vi "PS Set Rate.vi"(0 "VISA Resource Name":refnum<visa-resource-name>, 1 "Old Slew Rate":dbl format="%.1f", 2 "Slew Rate [A/S]":dbl format="%.1f", 3 "error In":errorcluster) -> (4 "Slew Rate Out [A/S]":dbl format="%.1f", 5 "dup VISA Resource Name":refnum<visa-resource-name>, 7 "Update?":bool, 8 "error Out":errorcluster)   [LabVIEW 2019]
uses:
  Serial Support VISA.llb/Serial Actions.ctl
  PS Comm Globals.vi
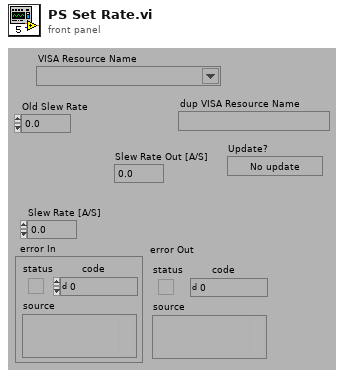
[diagram p1: front panel]
types:
  T1 = typedef "Serial Actions.ctl" = enum16{"Init", "Break", "Clear Buffer", "Write", "Read", "N Bytes", "Lock", "Unlock", "Close"}
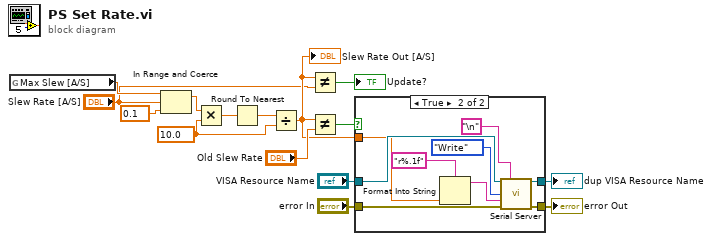
[diagram p0: block diagram]
diagram:
  w5 = 10.0 ("y")
  n1 = global read "PS Comm Globals.vi" "Max Slew [A/S]"() -> (w8:dbl)
  n2 = In Range and Coerce(upper limit=w8, x="Slew Rate [A/S]", lower limit=0.1 ("y")) -> (coerced(x)=w4:dbl)  [unwired: 1 out]
  n3 = Multiply(x=w4, y=w5) -> (x*y=w11:dbl)
  n4 = Round To Nearest(number=w11) -> (nearest integer value=w6:dbl)
  n5 = Divide(x=w6, y=w5) -> (x/y=w3:dbl)
  "Slew Rate Out [A/S]" <- w3
  n6 = Not Equal?(x=w3, y="Slew Rate [A/S]") -> (x != y?=→"Update?":bool)
  n7 = Not Equal?(x=w3, y="Old Slew Rate") -> (x != y?=w12:bool)
  n8 = case shown="True" w12 {
    tunnel: "error In" -> [w17 w26]
    tunnel: [w17 w25] -> w14
    tunnel: w3 -> [_ w19]
    tunnel: "VISA Resource Name" -> [w16 w20]
    tunnel: [w16 w18] -> w1
    frame False {
    }
    frame True {
      n9 = Format Into String(format string="r%.1f", w19) -> (resulting string=w22:string)  [unwired: 2 in, 1 out]
      n10 = call "Serial Server.vi"("VISA Resource Name"=w20, "EOT Chars (cr/lf)"="\n", "Action"=Serial_Actions."Write", "String To Send"=w22, "error in (no error)"=w26) -> ("dup VISA Resource Name"=w18:refnum<visa-resource-name>, "error out"=w25:errorcluster)  [unwired: 6 in, 3 out]
    }
  }
  "error Out" <- w14
  "dup VISA Resource Name" <- w1
